vi "test Get Channel Values.vi"(8 "error in (no error)":errorcluster, 11 "TestCase in":refnum<class "SLSC EDS System Tests.lvclass">) -> (0 "error out":errorcluster, 3 "TestCase out":refnum<class "SLSC EDS System Tests.lvclass">)   [LabVIEW 2015, in "SLSC EDS System Tests.lvclass"]
uses:
  SLSC EDS System Tests.lvclass
  <vilib>/NI Veristand/Execution/Workspace/NI VeriStand - Get Multiple Channel Values.vi
  <vilib>/addons/_JKI Toolkits/VI Tester/TestCase.llb/TestCase.lvclass
  <vilib>/NI VeriStand/Execution/Workspace/NI_VS Workspace ExecutionAPI.lvlib
panel:
  out "Measured Values":dbl[](array[numeric])=[3.0, 5.0]
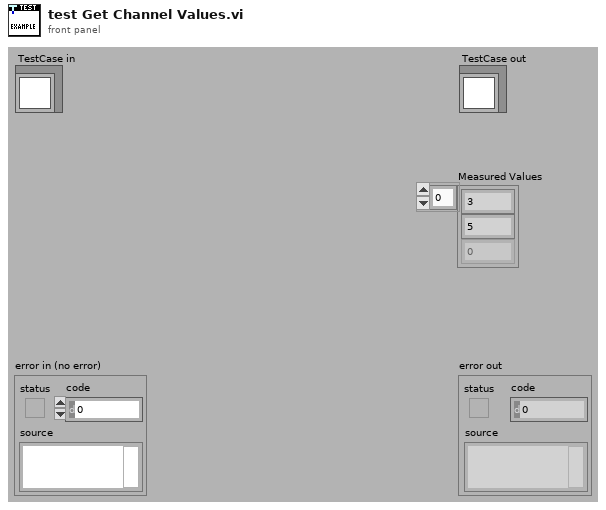
[diagram p1: front panel]
types:
  T1 = typedef "NI_VS Workspace ExecutionAPI.lvlib/WorkspaceAPI.ctl" = refnum<k24>
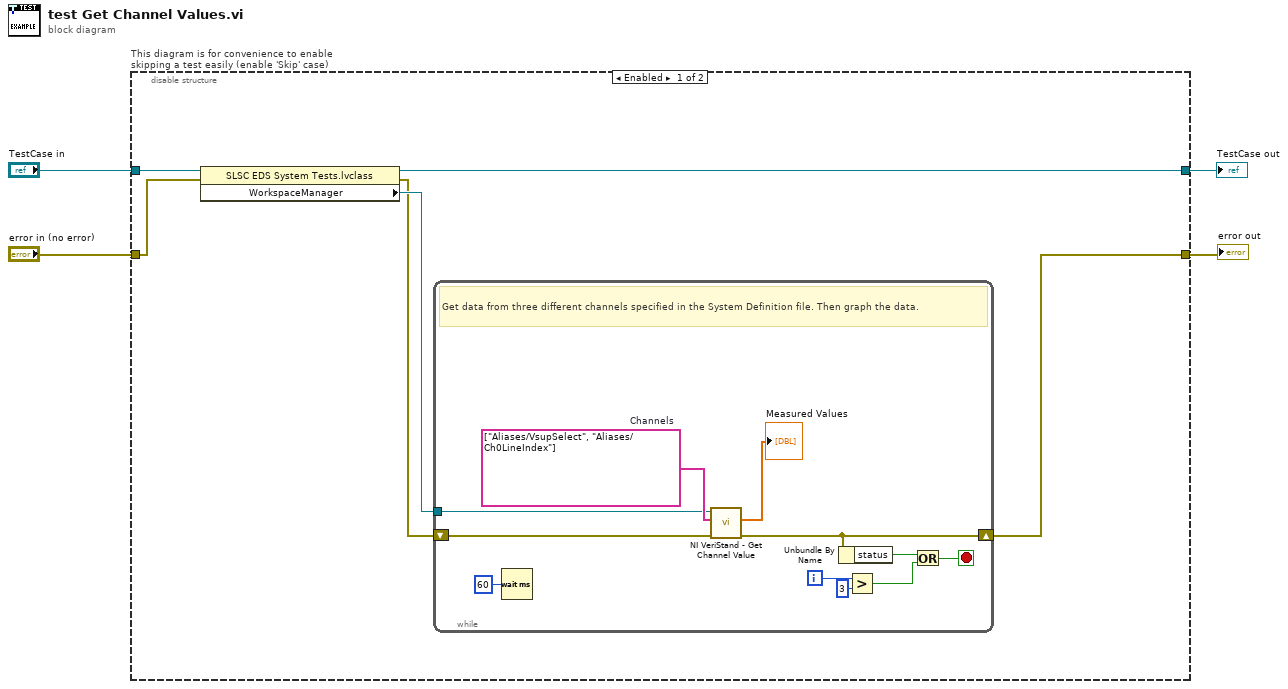
[diagram p0: block diagram]
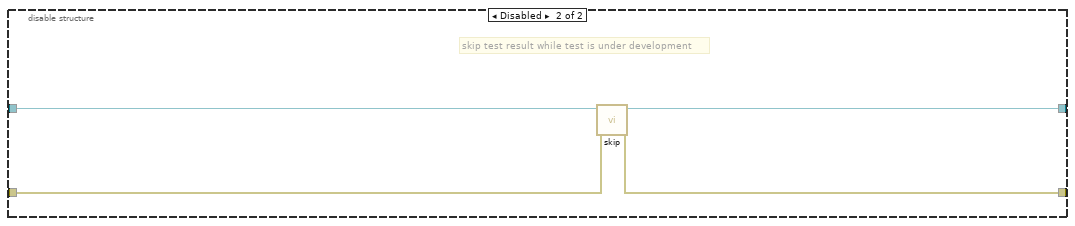
[diagram p2: hidden frame]
diagram:
  n1 = disable-structure "This diagram is for convenience to enable skipping a test easily (enable 'Skip' case)" shown="Enabled" {
    disable-tunnel: "TestCase in" -> [w9 w25]
    disable-tunnel: [w8 w23] -> w1
    disable-tunnel: [w10 w24] -> w3
    disable-tunnel: "error in (no error)" -> [w6 w22]
    frame Enabled {
      n2 = property class="SLSC EDS System Tests.lvclass"(reference=w9, error in=w6) -> (reference out=w8:refnum<class "SLSC EDS System Tests.lvclass">, error out=w5:errorcluster, "WorkspaceManager"=w7:T1)
      n3 = while {
        shift-right: [w18] -> w10
        shift-left: w5 -> [w19]
        tunnel: w7 -> [w11]
        i -> [w14]
        stop <- w21 stop-if-true
        w16 = string[] ["Aliases/VsupSelect", "Aliases/Ch0LineIndex"]  # Channels
        # "Get data from three different channels specified in the System Definition file. Then graph the data."
        n4 = Wait (ms)(milliseconds to wait=u32 60) -> ()  [unwired: 1 out]
        n5 = call-poly <vilib>:"NI VeriStand - Get Channel Value.vi"("error in (no error)"=w19, "Channels"=w16, "WorkspaceManager in"=w11) -> ("error out"=w18:errorcluster, "Values"=→"Measured Values":dbl[])  [unwired: 6 in, 1 out]
        n6 = Unbundle By Name(w18) -> ("status"=w20:bool)
        n7 = Greater?(x=w14, y=3) -> (0:w12:bool)
        n8 = Or(x=w20, y=w12) -> (x .or. y?=w21:bool)
      }
    }
    frame Disabled {
      # "skip test result while test is under development"
      n9 = call <vilib>:"skip.vi"("error in (no error)"=w22, "TestCase in"=w25) -> ("error out"=w24:errorcluster, "TestCase out"=w23:refnum<class "SLSC EDS System Tests.lvclass">)  [unwired: 8 in]
    }
  }
  "error out" <- w3
  "TestCase out" <- w1
